vi "jojo_original.vi"() -> ()   [LabVIEW 2021]
uses:
  <vilib>/numeric/Random Number (Range) U64.vi
  <vilib>/numeric/sub_Random U32.vi
panel:
  in  "Combo Box":string(combo)
  in  "File Name (include extension)":string
  out "error out":errorcluster
  out "Mixed Signal Graph 1":cluster{"Present (s)":dbl, "number":u64}[](graph)
  out "Mixed Signal Graph 2":cluster{"Present (s)":dbl, "number":u64}[](graph)
  out "Mixed Signal Graph 3":cluster{"Present (s)":dbl, "number":u64}[](graph)
  out "Mixed Signal Graph 5":T1(graph)
  out "Mixed Signal Graph 4":T2(graph)
  out "output cluster":T3
  out "Elapsed Time (s)":dbl format="%<%H:%M:%S\n%y/%m/%d>T"
  out "millisecond timer value":u32
  in  "stop":bool
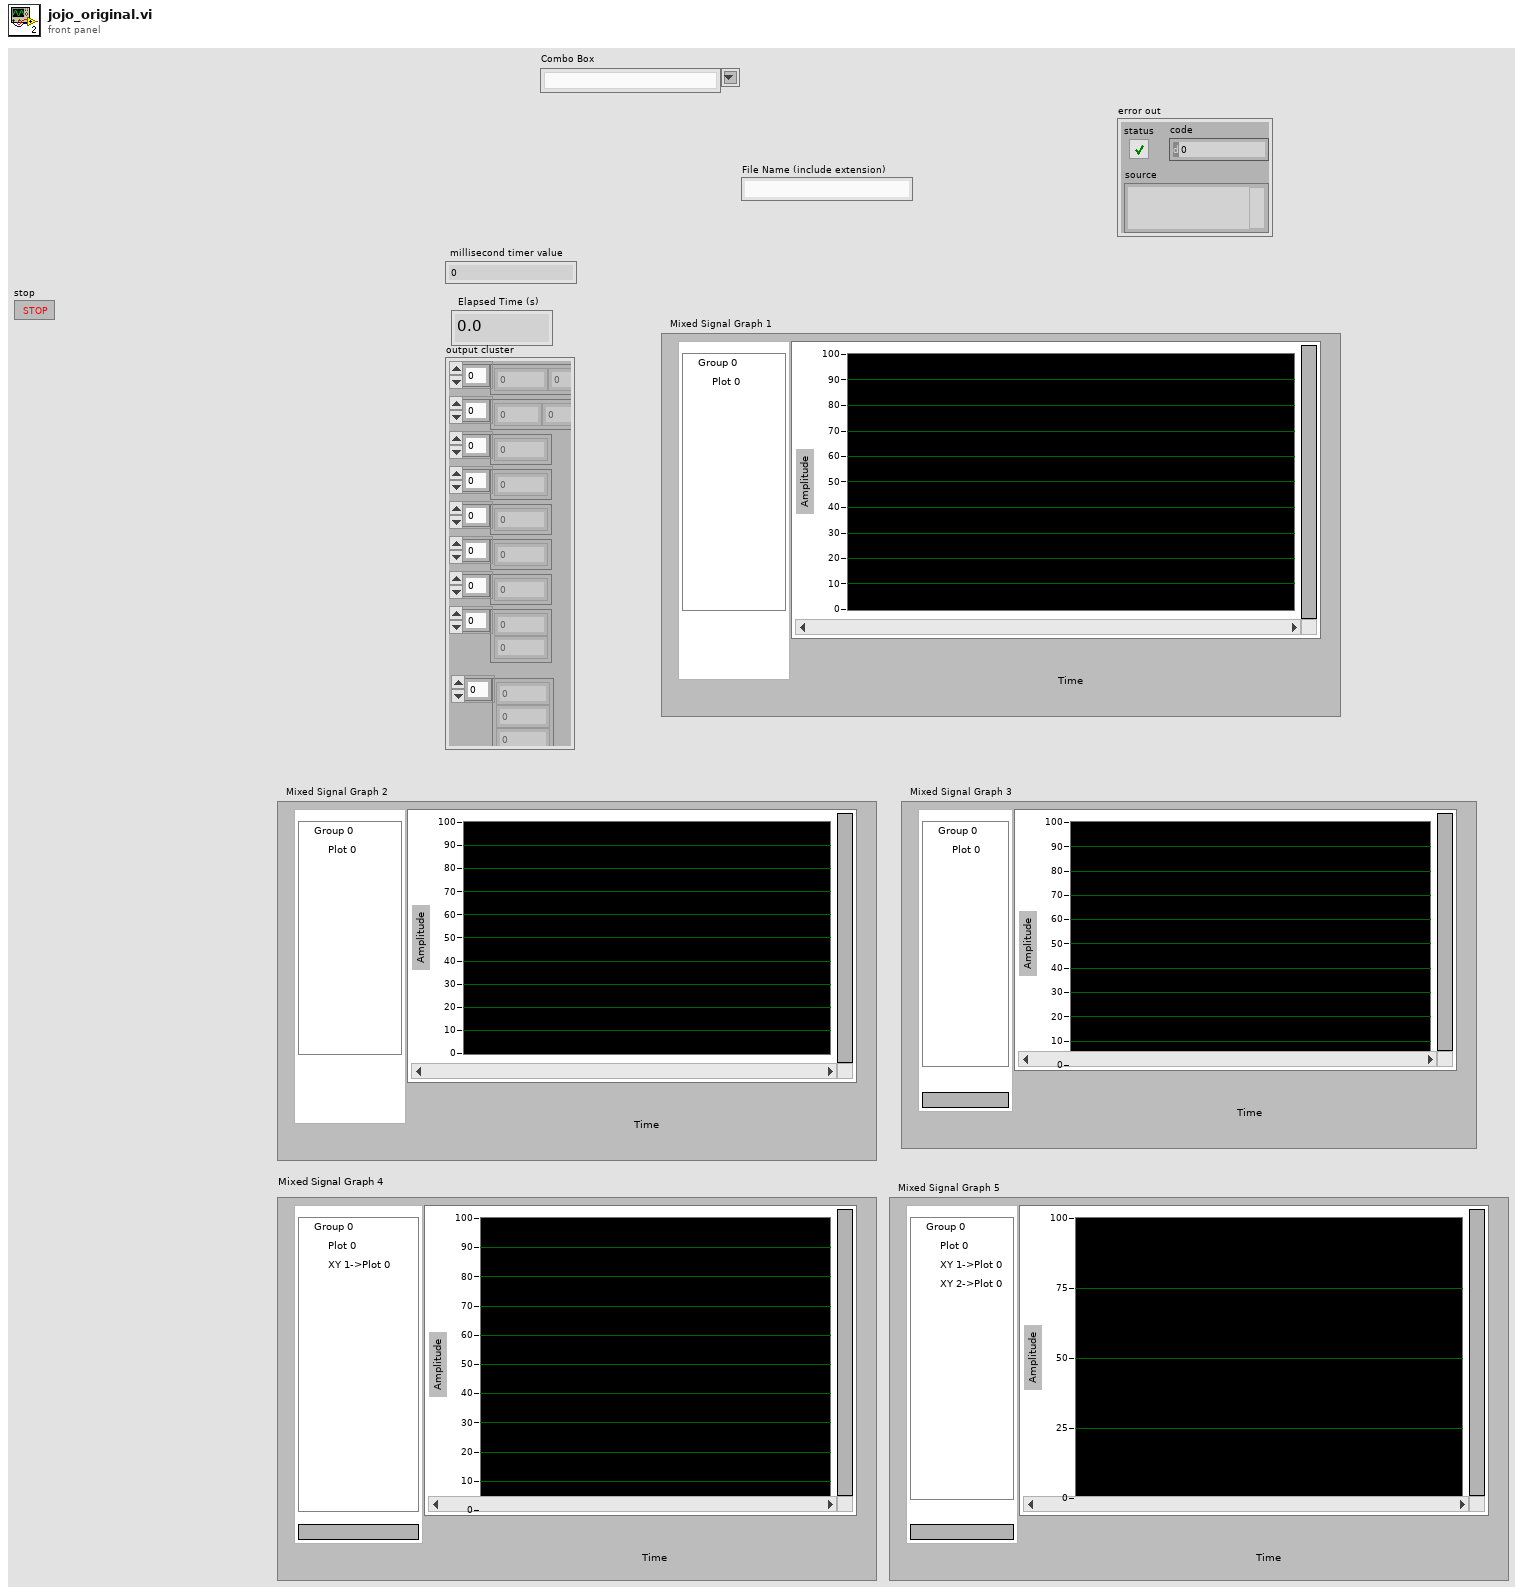
[diagram p1: front panel]
types:
  T1 = cluster{cluster{"Present (s)":dbl, "number":u64}[], cluster{"Present (s)":dbl, "number":u64}[], cluster{"Present (s)":dbl, "number":u64}[]}
  T2 = cluster{cluster{"Present (s)":dbl, "number":u64}[], cluster{"Present (s)":dbl, "number":u64}[]}
  T3 = cluster{u64[], u64[], u64[], u64[], u64[], u64[], u64[], u64[], dbl[]}
  T4 = enum16{"open", "replace", "create", "open or create", "replace or create", "replace or create with confirmation"}
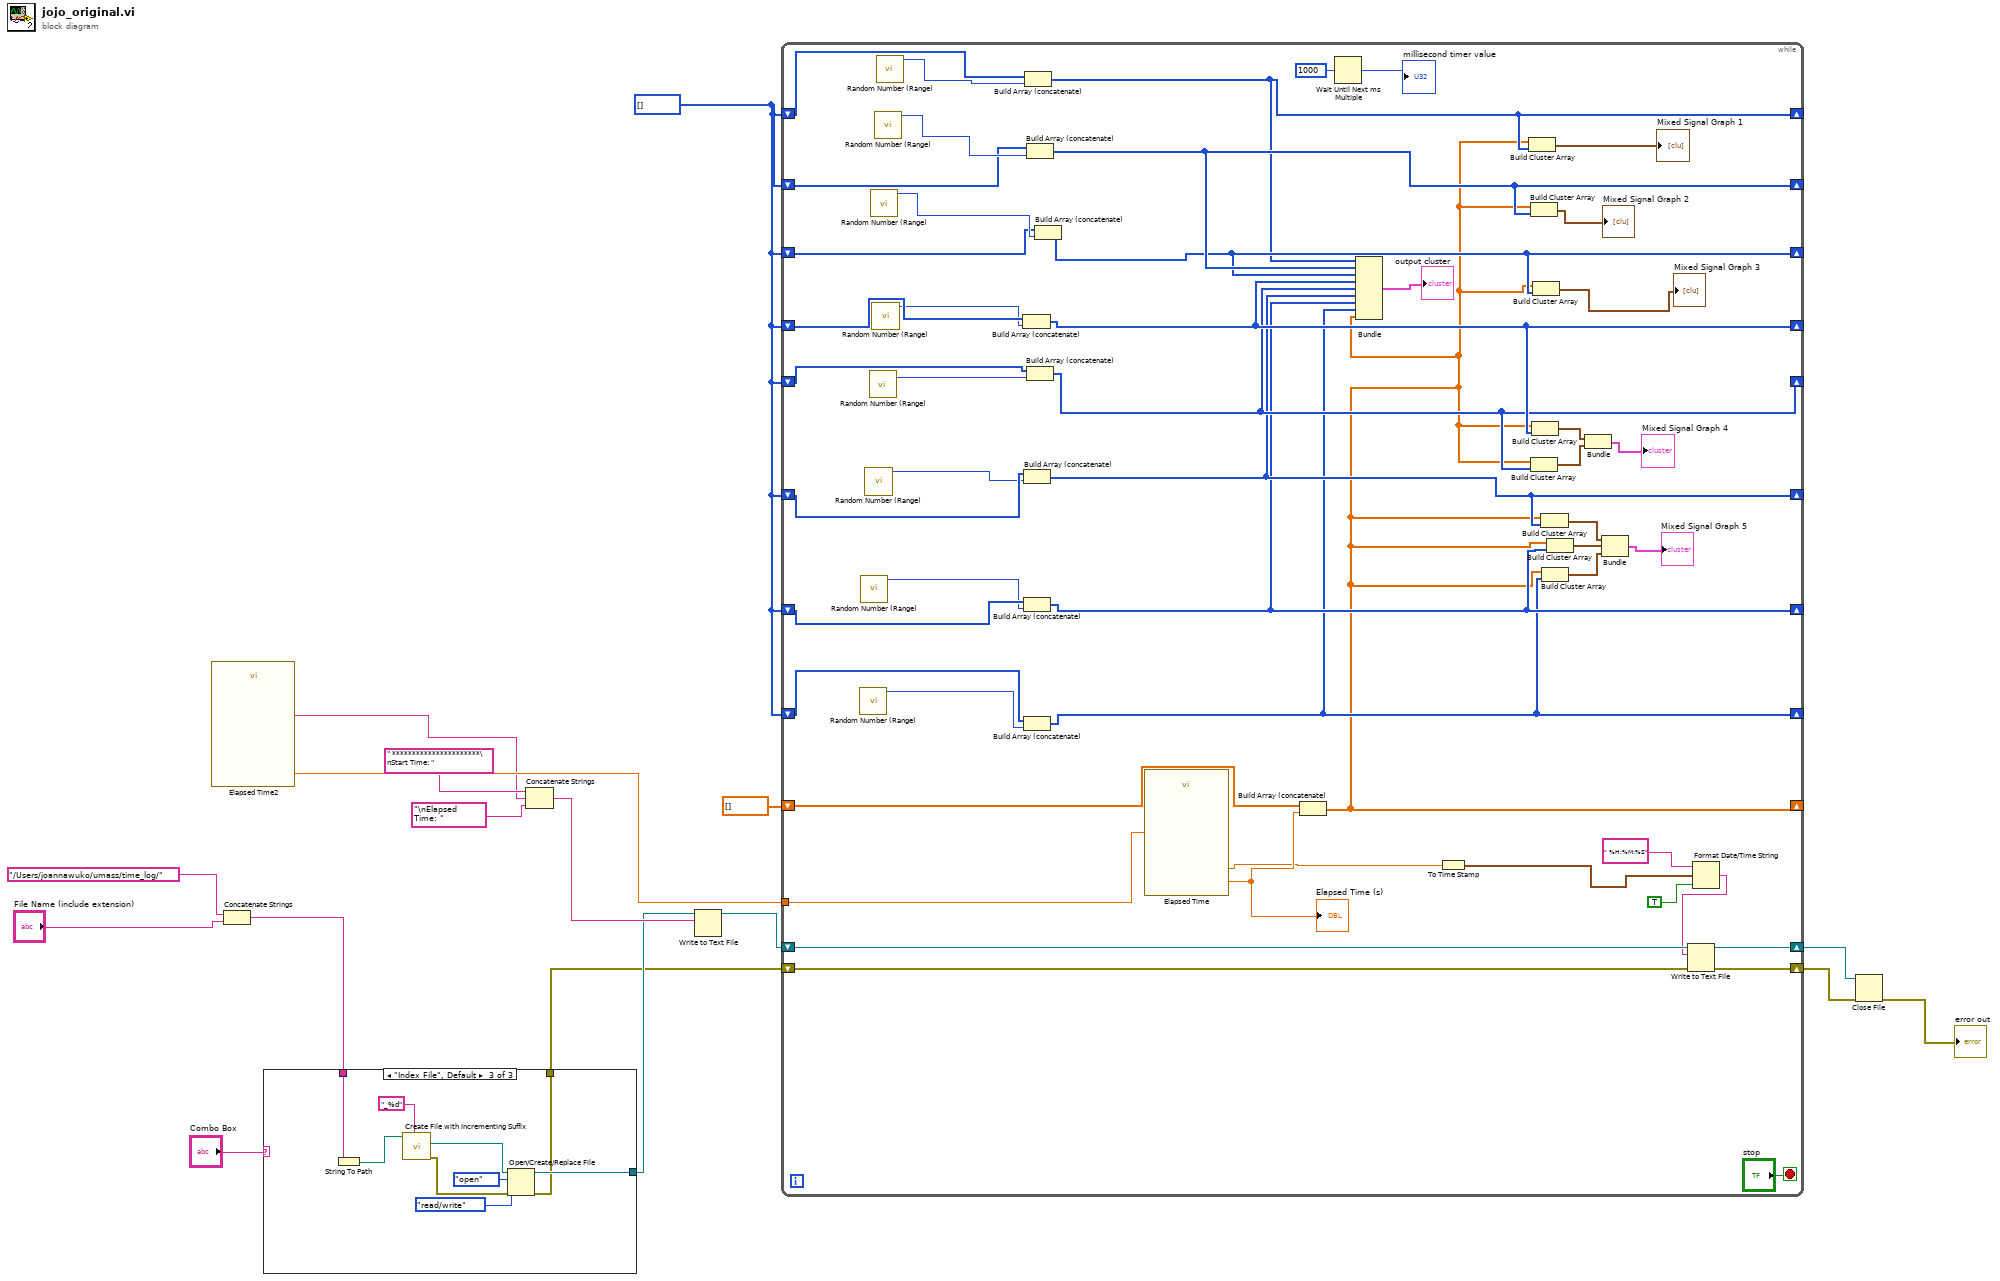
[diagram p0: block diagram]
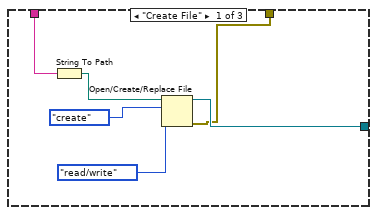
[diagram p2: hidden frame]
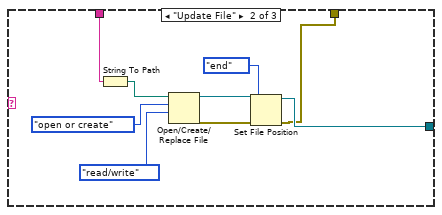
[diagram p3: hidden frame]
diagram:
  w15 = u64[] []
  n1 = call "Elapsed Time2"() -> ("Start Time Text"=w10:string, "Present (s)"=w17:dbl)  [unwired: 12 in, 6 out]
  n2 = Concatenate Strings("/Users/joannawuko/umass/time_log/" ("string"), "File Name (include extension)") -> (w3:string)
  n3 = case shown="\"Index File\", Default" "Combo Box" {
    tunnel: [w23 w29 w37] -> w5
    tunnel: [w22 w27 w36] -> w4
    tunnel: w3 -> [w19 w32 w35]
    frame "Create File" {
      n4 = String To Path(string=w19) -> (path=w18:path)
      n5 = Open/Create/Replace File(file path (use dialog)=w18, operation (0:open)=T4."create", access (0:read/write)=enum16{"read/write", "read-only", "write-only"}."read/write") -> (refnum out=w23:refnum<file>, error out=w22:errorcluster)  [unwired: 3 in, 1 out]
    }
    frame "Update File" {
      n6 = String To Path(string=w32) -> (path=w31:path)
      n7 = Open/Create/Replace File(file path (use dialog)=w31, operation (0:open)=T4."open or create", access (0:read/write)=enum16{"read/write", "read-only", "write-only"}."read/write") -> (refnum out=w30:refnum<file>, error out=w26:errorcluster)  [unwired: 3 in, 1 out]
      n8 = Set File Position(refnum=w30, from (0:start)=enum16{"start", "end", "current"}."end", error in=w26) -> (refnum out=w29:refnum<file>, error out=w27:errorcluster)  [unwired: 1 in]
    }
    frame "Index File", Default {
      n9 = String To Path(string=w35) -> (path=w34:path)
      n10 = call <vilib>:"Create File with Incrementing Suffix.vi"("format string (\" (%d)\")"="_%d" ("format string (\" (%d)\")"), "file path"=w34) -> ("error out"=w33:errorcluster, "actual path"=w41:path)  [unwired: 7 in, 1 out]
      n11 = Open/Create/Replace File(file path (use dialog)=w41, error in=w33, operation (0:open)=T4."open", access (0:read/write)=enum16{"read/write", "read-only", "write-only"}."read/write") -> (refnum out=w37:refnum<file>, error out=w36:errorcluster)  [unwired: 2 in, 1 out]
    }
  }
  n12 = Concatenate Strings(" **********************\nStart Time: ", w10, "\nElapsed Time: ") -> (w9:string)
  n13 = Write to Text File(file (use dialog)=w5, text=w9) -> (refnum out=w8:refnum<file>)  [unwired: 2 in, 2 out]
  n14 = while {
    shift-right: [w69] -> _
    shift-left: w15 -> [w71]
    shift-right: [w70] -> _
    shift-left: w15 -> [w72]
    shift-right: [w68] -> _
    shift-left: w15 -> [w73]
    shift-right: [w65] -> _
    shift-left: w15 -> [w89]
    shift-right: [w64] -> _
    shift-left: w15 -> [w87]
    shift-right: [w63] -> _
    shift-left: w15 -> [w85]
    shift-right: [w62] -> _
    shift-left: w15 -> [w83]
    shift-right: [w61] -> _
    shift-left: w15 -> [w81]
    tunnel: w17 -> [w79]
    shift-right: [w57] -> _
    shift-left: dbl[] [] -> [w78]
    shift-right: [w51] -> w14
    shift-left: w8 -> [w48]
    shift-right: [w50] -> w13
    shift-left: w4 -> [w49]
    stop <- "stop" stop-if-true
    n15 = call-poly <vilib>:"Random Number (Range).vi"() -> ("number"=w80:u64)  [unwired: 11 in]
    n16 = call-poly <vilib>:"Random Number (Range).vi"() -> ("number"=w82:u64)  [unwired: 11 in]
    n17 = call-poly <vilib>:"Random Number (Range).vi"() -> ("number"=w84:u64)  [unwired: 11 in]
    n18 = call-poly <vilib>:"Random Number (Range).vi"() -> ("number"=w86:u64)  [unwired: 11 in]
    n19 = call-poly <vilib>:"Random Number (Range).vi"() -> ("number"=w74:u64)  [unwired: 11 in]
    n20 = call-poly <vilib>:"Random Number (Range).vi"() -> ("number"=w88:u64)  [unwired: 11 in]
    n21 = call-poly <vilib>:"Random Number (Range).vi"() -> ("number"=w75:u64)  [unwired: 11 in]
    n22 = call-poly <vilib>:"Random Number (Range).vi"() -> ("number"=w76:u64)  [unwired: 11 in]
    n23 = Build Array (concatenate)(w89, w88) -> (w65:u64[])
    n24 = Build Array (concatenate)(w85, w84) -> (w63:u64[])
    n25 = Build Array (concatenate)(w83, w82) -> (w62:u64[])
    n26 = Build Array (concatenate)(w81, w80) -> (w61:u64[])
    n27 = Build Array (concatenate)(w73, w76) -> (w68:u64[])
    n28 = Build Array (concatenate)(w72, w75) -> (w70:u64[])
    n29 = Build Array (concatenate)(w87, w86) -> (w64:u64[])
    n30 = Build Array (concatenate)(w71, w74) -> (w69:u64[])
    n31 = call "Elapsed Time"("Set Start Time (s)"=w79) -> ("Present (s)"=w47:dbl, "Elapsed Time (s)"=w46:dbl)  [unwired: 11 in, 6 out]
    "Elapsed Time (s)" <- w47
    n32 = Build Array (concatenate)(w78, w47) -> (w57:dbl[])
    n33 = Wait Until Next ms Multiple(millisecond multiple=u32 1000) -> (millisecond timer value=→"millisecond timer value":u32)
    n34 = Bundle(w68, w70, w69, w65, w64, w63, w62, w61, w57) -> (→"output cluster":T3)  [unwired: 1 in]
    n35 = To Time Stamp(1:w46) -> (0:w42:timestamp)
    n36 = Build Cluster Array(w57, w68) -> (→"Mixed Signal Graph 1":cluster{"Present (s)":dbl, "number":u64}[])
    n37 = Build Cluster Array(w57, w70) -> (→"Mixed Signal Graph 2":cluster{"Present (s)":dbl, "number":u64}[])
    n38 = Build Cluster Array(w57, w64) -> (w66:cluster{"Present (s)":dbl, "number":u64}[])
    n39 = Build Cluster Array(w57, w65) -> (w67:cluster{"Present (s)":dbl, "number":u64}[])
    n40 = Build Cluster Array(w57, w69) -> (→"Mixed Signal Graph 3":cluster{"Present (s)":dbl, "number":u64}[])
    n41 = Build Cluster Array(w57, w63) -> (w60:cluster{"Present (s)":dbl, "number":u64}[])
    n42 = Build Cluster Array(w57, w61) -> (w58:cluster{"Present (s)":dbl, "number":u64}[])
    n43 = Build Cluster Array(w57, w62) -> (w59:cluster{"Present (s)":dbl, "number":u64}[])
    n44 = Bundle(w67, w66) -> (→"Mixed Signal Graph 4":T2)  [unwired: 1 in]
    n45 = Bundle(w60, w59, w58) -> (→"Mixed Signal Graph 5":T1)  [unwired: 1 in]
    n46 = Format Date/Time String(time format string (%c)=" %H:%M:%S", seconds (now)=w42, UTC format=TRUE) -> (date/time string=w45:string)
    n47 = Write to Text File(file (use dialog)=w48, text=w45, error in=w49) -> (refnum out=w51:refnum<file>, error out=w50:errorcluster)  [unwired: 1 in, 1 out]
  }
  n48 = Close File(refnum=w14, error in=w13) -> (error out=→"error out":errorcluster)  [unwired: 1 out]
